vi "addToQueue.vi"(2 "Message":string, 3 "ROS_Master":refnum<class "ROS_Master.lvclass">) -> ()   [LabVIEW 2013, in "ROS_Master.lvclass"]
uses:
  <userlib>/ROS_Master/ROS_Master.lvclass
  <userlib>/ROS_Master/ROS_Master.lvclass/ROS_Master.ctl
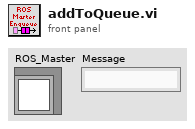
[diagram p1: front panel]
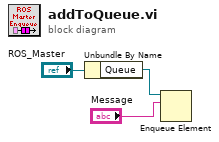
[diagram p0: block diagram]
diagram:
  n1 = Unbundle By Name("ROS_Master") -> ("Queue"=w2:refnum<queue>)
  n2 = Enqueue Element(queue=w2, element="Message") -> ()  [unwired: 2 in, 3 out]
